vi "Read output L.vi"(11 "PID_OL_AM in":refnum<class "PID_OL_AM.lvclass">) -> (2 "output L":dbl=-100.0 format="%.2f", 3 "PID_OL_AM out":refnum<class "PID_OL_AM.lvclass">)   [LabVIEW 2019, in "control.lvlib" / "PID_OL_AM.lvclass"]
uses:
  PID_OL_AM.lvclass
  PID_OL_AM.lvclass/PID_OL_AM.ctl
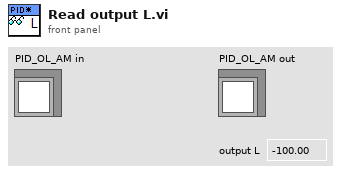
[diagram p1: front panel]
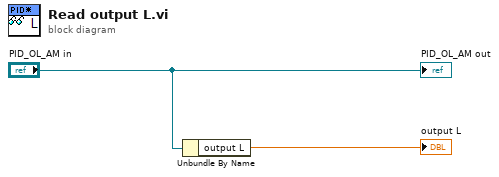
[diagram p0: block diagram]
diagram:
  n1 = Unbundle By Name("PID_OL_AM in") -> ("output L"=→"output L":dbl)
  "PID_OL_AM out" <- "PID_OL_AM in"
